vi "Has Node.vi"(8 "error in (no error)":errorcluster, 10 "Path":string, 11 "Tree in":refnum<class "Tree.lvclass">) -> (0 "error out":errorcluster, 1 "Has Node":bool, 3 "Tree out":refnum<class "Tree.lvclass">)   [LabVIEW 2015, in "MDSplus.lvlib" / "Tree.lvclass"]
doc: "Return TreeNode for the data item corresponding to the passed pathname."
uses:
  <vilib>/MDSplus/Classes/Tree_Class/Tree.lvclass
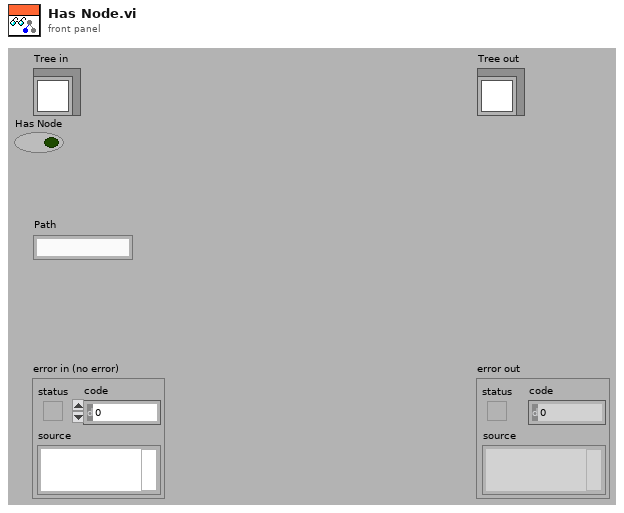
[diagram p1: front panel]
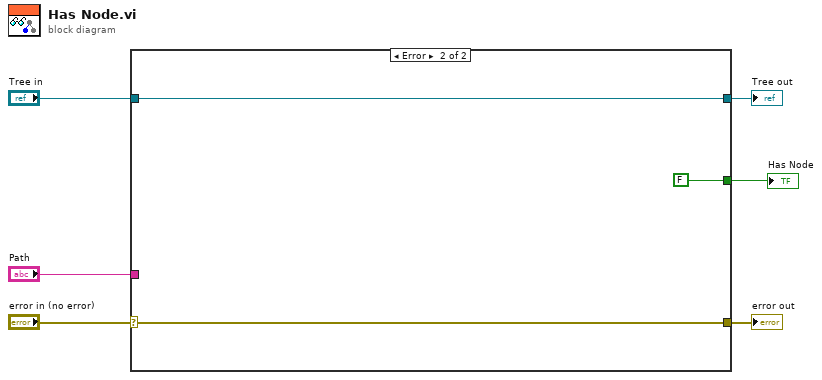
[diagram p0: block diagram]
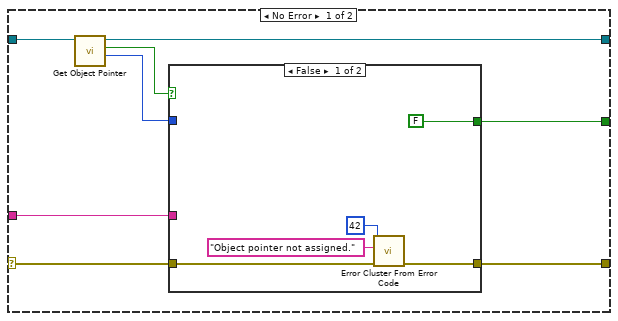
[diagram p2: hidden frame]
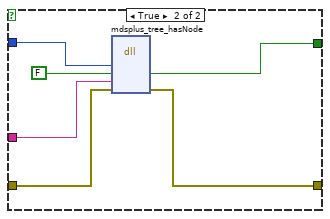
[diagram p3: hidden frame]
diagram:
  n1 = case shown="Error" "error in (no error)" {
    selector: "error in (no error)" -> [w9 w28]
    tunnel: [w8 w28] -> w5
    tunnel: [w13 w27] -> w3
    tunnel: "Tree in" -> [w14 w27]
    tunnel: "Path" -> [w12 _]
    tunnel: [w7 FALSE] -> w1
    frame No Error {
      n2 = call-dynamic "Get Object Pointer.vi"("Tree in"=w14) -> ("Object Pointer"=w10:i64, "Assigned object pointer?"=w11:bool, "Tree out"=w13:refnum<class "Tree.lvclass">)  [unwired: 8 in]
      n3 = case shown="False" w11 {
        tunnel: w12 -> [_ w25]
        tunnel: w10 -> [_ w24]
        tunnel: w9 -> [w17 w23]
        tunnel: [w16 w22] -> w8
        tunnel: [FALSE w20] -> w7
        frame False {
          n4 = call <vilib>:"Error Cluster From Error Code.vi"("error in (no error)"=w17, "error message (\"\")"="Object pointer not assigned." ("error message (\"\")"), "error code (0)"=42) -> ("error out"=w16:errorcluster)  [unwired: 6 in]
        }
        frame True {
          n5 = dll-call lib="MDSobjectsLVShr" fn="mdsplus_tree_hasNode"("lvTreePtr"=w24, "lvTreeHasNodeOut"=FALSE, "pathIn"=w25, "error"=w23) -> ("lvTreeHasNodeOut"=w20:bool, "error"=w22:errorcluster)  [unwired: 6 in, 2 out]
        }
      }
    }
    frame Error {
    }
  }
  "error out" <- w5
  "Tree out" <- w3
  "Has Node" <- w1
